vi "ElevatorStateControl.vi"(9 "Elevator State":string) -> (1 "Elevator State Out":string, 2 "Target Elevator Position":dbl, 4 "Target Vacuum Pump Power":dbl)   [LabVIEW 2018]
uses:
  Inputs_DriverStation.vi
  SensorReadings.vi
  RobotStates.vi
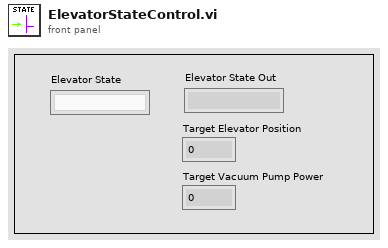
[diagram p1: front panel]
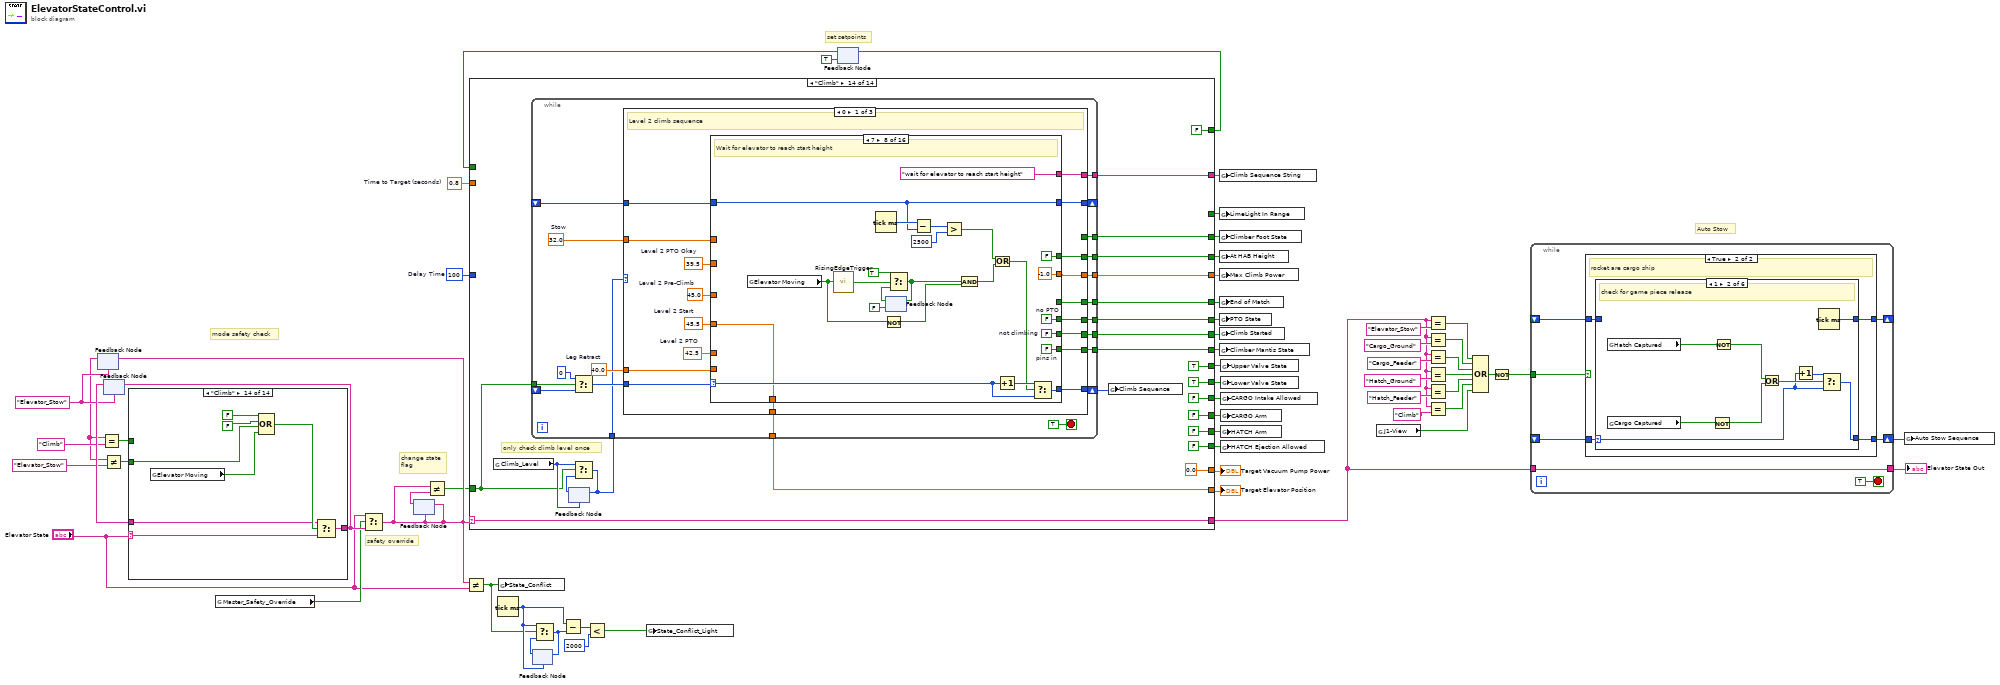
[diagram p0: block diagram]
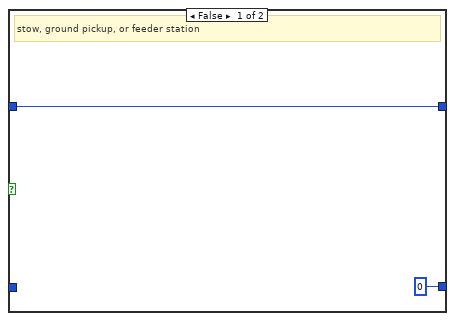
[diagram p2: hidden frame]
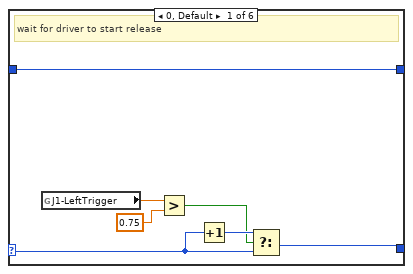
[diagram p3: hidden frame]
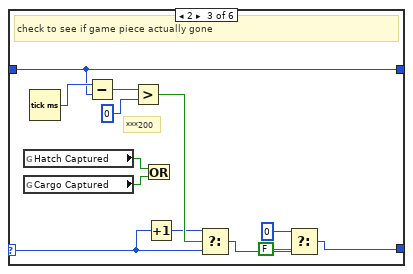
[diagram p4: hidden frame]
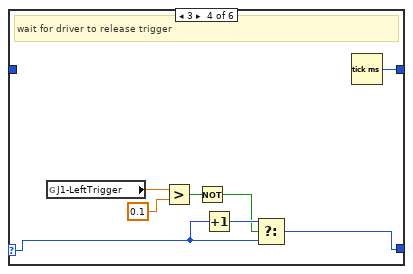
[diagram p5: hidden frame]
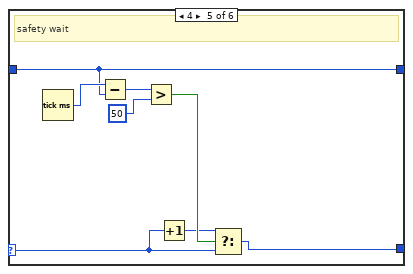
[diagram p6: hidden frame]
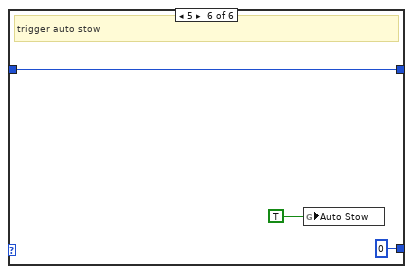
[diagram p7: hidden frame]
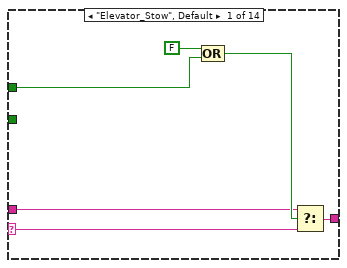
[diagram p8: hidden frame]
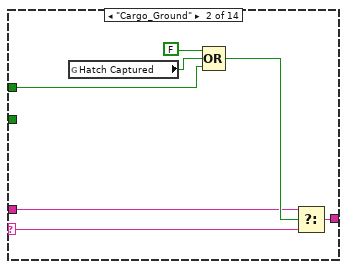
[diagram p9: hidden frame]
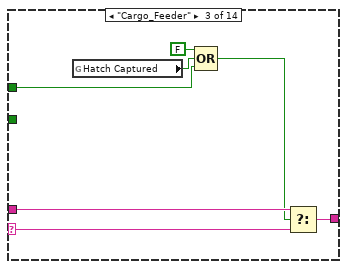
[diagram p10: hidden frame]
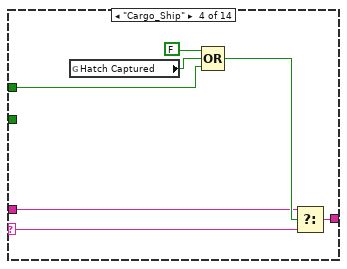
[diagram p11: hidden frame]
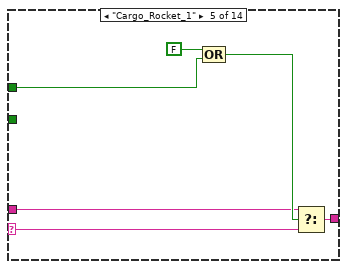
[diagram p12: hidden frame]
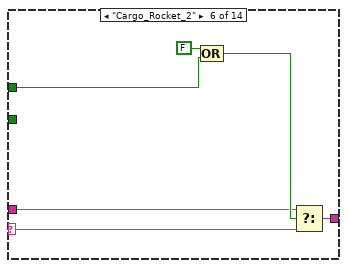
[diagram p13: hidden frame]
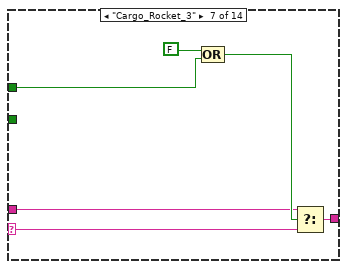
[diagram p14: hidden frame]
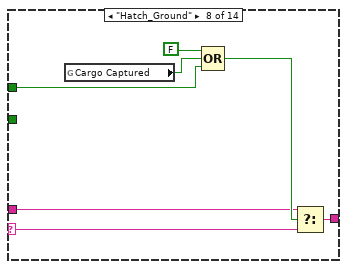
[diagram p15: hidden frame]
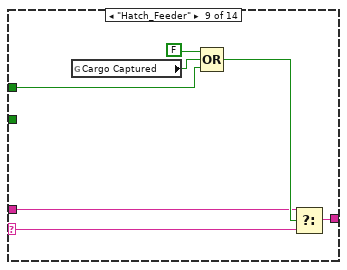
[diagram p16: hidden frame]
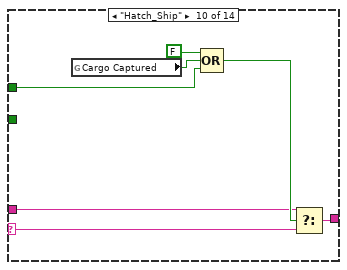
[diagram p17: hidden frame]
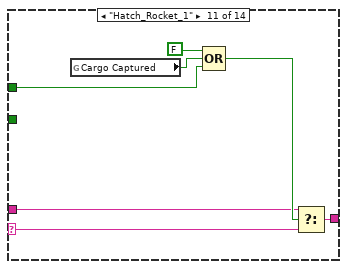
[diagram p18: hidden frame]
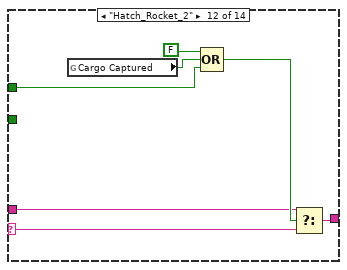
[diagram p19: hidden frame]
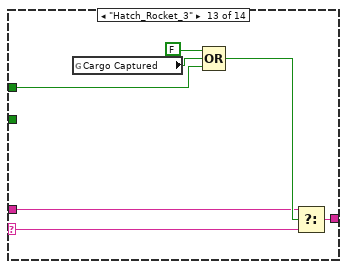
[diagram p20: hidden frame]
diagram:
  w3 = u32 100  # Delay Time
  w4 = 0.8  # Time to Target (seconds)
  w46 = "Elevator_Stow" ("Elevator State")
  # "change state\nflag"
  # "Auto Stow"
  # "safety override"
  # "mode safety check"
  # "set setpoints"
  n1 = feedback #1(w46) -> (w11:string)
  n2 = Equal?(x=w11, y="Climb") -> (x = y?=w47:bool)
  n3 = feedback #2(w46) -> (w49:string)
  n4 = Not Equal?(x=w11, y="Elevator_Stow") -> (x != y?=w10:bool)
  n5 = case shown="\"Climb\"" "Elevator State" {
    selector: "Elevator State" -> [w62 w69 w80 w83 w89 w95 w102 w108 w115 w122 w129 w136 w144 w152]
    tunnel: [w64 w71 w79 w85 w91 w97 w103 w110 w117 w124 w131 w138 w145 w153] -> w54
    tunnel: w49 -> [w63 w70 w78 w84 w90 w96 w101 w109 w116 w123 w130 w137 w143 w151]
    tunnel: w47 -> [w61 w67 w74 w81 w88 w94 w100 w106 w113 w120 w127 w134 w141 _]
    tunnel: w10 -> [_ _ _ _ _ _ _ _ _ _ _ _ _ w150]
    frame "Elevator_Stow", Default {
      n6 = Compound Arithmetic op=OR(FALSE, w61) -> (w65:bool)
      n7 = Select(t=w63, s=w65, f=w62) -> (s? t:f=w64:string)
    }
    frame "Cargo_Ground" {
      n8 = global read "SensorReadings.vi" "Hatch Captured"() -> (w68:bool)
      n9 = Compound Arithmetic op=OR(FALSE, w68, w67) -> (w72:bool)
      n10 = Select(t=w70, s=w72, f=w69) -> (s? t:f=w71:string)
    }
    frame "Cargo_Feeder" {
      n11 = global read "SensorReadings.vi" "Hatch Captured"() -> (w75:bool)
      n12 = Compound Arithmetic op=OR(FALSE, w75, w74) -> (w76:bool)
      n13 = Select(t=w78, s=w76, f=w80) -> (s? t:f=w79:string)
    }
    frame "Cargo_Ship" {
      n14 = global read "SensorReadings.vi" "Hatch Captured"() -> (w82:bool)
      n15 = Compound Arithmetic op=OR(FALSE, w82, w81) -> (w86:bool)
      n16 = Select(t=w84, s=w86, f=w83) -> (s? t:f=w85:string)
    }
    frame "Cargo_Rocket_1" {
      n17 = Compound Arithmetic op=OR(FALSE, w88) -> (w92:bool)
      n18 = Select(t=w90, s=w92, f=w89) -> (s? t:f=w91:string)
    }
    frame "Cargo_Rocket_2" {
      n19 = Compound Arithmetic op=OR(FALSE, w94) -> (w98:bool)
      n20 = Select(t=w96, s=w98, f=w95) -> (s? t:f=w97:string)
    }
    frame "Cargo_Rocket_3" {
      n21 = Compound Arithmetic op=OR(FALSE, w100) -> (w104:bool)
      n22 = Select(t=w101, s=w104, f=w102) -> (s? t:f=w103:string)
    }
    frame "Hatch_Ground" {
      n23 = global read "SensorReadings.vi" "Cargo Captured"() -> (w107:bool)
      n24 = Compound Arithmetic op=OR(FALSE, w107, w106) -> (w111:bool)
      n25 = Select(t=w109, s=w111, f=w108) -> (s? t:f=w110:string)
    }
    frame "Hatch_Feeder" {
      n26 = global read "SensorReadings.vi" "Cargo Captured"() -> (w114:bool)
      n27 = Compound Arithmetic op=OR(FALSE, w114, w113) -> (w118:bool)
      n28 = Select(t=w116, s=w118, f=w115) -> (s? t:f=w117:string)
    }
    frame "Hatch_Ship" {
      n29 = global read "SensorReadings.vi" "Cargo Captured"() -> (w121:bool)
      n30 = Compound Arithmetic op=OR(FALSE, w121, w120) -> (w125:bool)
      n31 = Select(t=w123, s=w125, f=w122) -> (s? t:f=w124:string)
    }
    frame "Hatch_Rocket_1" {
      n32 = global read "SensorReadings.vi" "Cargo Captured"() -> (w128:bool)
      n33 = Compound Arithmetic op=OR(FALSE, w128, w127) -> (w132:bool)
      n34 = Select(t=w130, s=w132, f=w129) -> (s? t:f=w131:string)
    }
    frame "Hatch_Rocket_2" {
      n35 = global read "SensorReadings.vi" "Cargo Captured"() -> (w135:bool)
      n36 = Compound Arithmetic op=OR(FALSE, w135, w134) -> (w139:bool)
      n37 = Select(t=w137, s=w139, f=w136) -> (s? t:f=w138:string)
    }
    frame "Hatch_Rocket_3" {
      n38 = global read "SensorReadings.vi" "Cargo Captured"() -> (w142:bool)
      n39 = Compound Arithmetic op=OR(FALSE, w142, w141) -> (w146:bool)
      n40 = Select(t=w143, s=w146, f=w144) -> (s? t:f=w145:string)
    }
    frame "Climb" {
      n41 = global read "RobotStates.vi" "Elevator Moving"() -> (w149:bool)
      n42 = Compound Arithmetic op=OR(FALSE, FALSE ("Cargo Captured"), w150, w149) -> (w154:bool)
      n43 = Select(t=w151, s=w154, f=w152) -> (s? t:f=w153:string)
    }
  }
  n44 = feedback-in #2(w54) -> ()
  n45 = global read "Inputs_DriverStation.vi" "Master_Safety_Override"() -> (w53:bool)
  n46 = Select(t="Elevator State", s=w53, f=w54) -> (s? t:f=w16:string)
  n47 = feedback-in #1(w16) -> ()
  n48 = feedback-in #3(w16) -> ()
  n49 = feedback #3(w16) -> (w17:string)
  n50 = Not Equal?(x=w16, y=w17) -> (x != y?=w15:bool)
  n51 = Not Equal?(x=w16, y="Elevator State") -> (x != y?=w22:bool)
  n52 = Tick Count (ms)() -> (millisecond timer value=w26:u32)
  n53 = global write "RobotStates.vi" "State_Conflict"(w22) -> ()
  n54 = feedback #4(w26) -> (w27:u32)
  n55 = Select(t=w26, s=w22, f=w27) -> (s? t:f=w25:u32)
  n56 = feedback-in #4(w25) -> ()
  n57 = Subtract(x=w26, y=w25) -> (x-y=w24:u32)
  n58 = Less?(x=w24, y=u32 2000) -> (x < y?=w21:bool)
  n59 = global write "RobotStates.vi" "State_Conflict_Light"(w21) -> ()
  n60 = feedback #5(TRUE) -> (w19:bool)
  n61 = case shown="\"Climb\"" w16 {
    selector: w16 -> [w179 w194 w234 w252 w293 w315 w337 w351 w413 w454 w495 w510 w525 w550]
    tunnel: [FALSE TRUE TRUE TRUE TRUE TRUE TRUE FALSE FALSE FALSE FALSE FALSE FALSE FALSE] -> w60
    tunnel: [w179 w194 w234 w252 w293 w315 w337 w351 w413 w454 w495 w510 w525 w550] -> w29
    tunnel: [w157 FALSE w197 w235 TRUE w296 w319 FALSE FALSE FALSE FALSE FALSE FALSE FALSE] -> w59
    tunnel: [w178 32.0 w204 w236 w279 w300 w317 32.0 w378 w440 w481 61.5 91.0 w536] -> w58
    tunnel: [FALSE FALSE FALSE FALSE FALSE FALSE FALSE TRUE w382 TRUE TRUE TRUE TRUE FALSE] -> w57
    tunnel: [w170 0.0 0.0 0.0 0.0 0.0 0.0 w347 w411 w452 w493 w506 w521 0.0 ("Vacuum_Pump")] -> w55
    tunnel: [FALSE FALSE FALSE FALSE FALSE FALSE FALSE TRUE TRUE TRUE TRUE TRUE TRUE FALSE] -> w56
    tunnel: [TRUE TRUE TRUE TRUE TRUE TRUE TRUE TRUE FALSE FALSE FALSE FALSE FALSE TRUE] -> w52
    tunnel: [TRUE TRUE TRUE TRUE TRUE TRUE TRUE FALSE TRUE TRUE TRUE TRUE TRUE TRUE] -> w51
    tunnel: [FALSE FALSE FALSE FALSE FALSE FALSE FALSE FALSE FALSE FALSE FALSE FALSE FALSE w539] -> w1
    tunnel: [w168 FALSE FALSE FALSE FALSE FALSE FALSE FALSE FALSE FALSE FALSE FALSE FALSE FALSE] -> w20
    tunnel: w19 -> [w164 _ _ _ _ _ _ _ _ _ _ _ _ _]
    tunnel: w15 -> [_ _ w212 _ _ _ _ _ w384 _ _ _ _ w538]
    tunnel: [w167 w184 w203 w244 w284 w307 w329 w342 w390 w447 w488 w501 w516 w535] -> w14
    tunnel: [w166 w183 w202 w243 w283 w306 w328 w341 w389 w446 w487 w500 w515 w534] -> w13
    tunnel: [FALSE FALSE FALSE FALSE FALSE FALSE FALSE FALSE FALSE FALSE FALSE FALSE FALSE w533] -> w9
    tunnel: [_ _ _ _ _ _ _ _ _ _ _ _ _ w531] -> w8
    tunnel: [-1.0 ("y") -1.0 ("y") -1.0 ("y") -1.0 ("y") -1.0 ("y") -1.0 ("y") -1.0 ("y") -1.0 ("y") -1.0 ("y") -1.0 ("y") -1.0 ("y") -1.0 ("y") -1.0 ("y") w530] -> w7
    tunnel: [_ _ _ _ _ _ _ _ _ _ _ _ _ w529] -> w6
    tunnel: [_ _ _ _ w271 _ _ _ w371 w433 w474 _ _ _] -> w5
    tunnel: w4 -> [_ _ _ _ w269 _ _ _ w369 w432 w472 _ _ _]
    tunnel: w3 -> [_ _ _ _ w270 _ _ _ w370 w431 w473 _ _ _]
    tunnel: [_ _ _ _ _ _ _ _ _ _ _ _ _ w528] -> w2
    frame "Elevator_Stow", Default {
      w166 = FALSE  # no PTO
      w167 = FALSE  # not climbing
      w178 = 30.0  # below 34.5 to ensure reset
      n62 = global read "Inputs_DriverStation.vi" "Reinit_Stow_Vacuum"() -> (w161:bool)
      n63 = global read "Inputs_DriverStation.vi" "Vacuum_Pump"() -> (w172:dbl)
      n64 = global read "RobotStates.vi" "Autopilot"() -> (w160:bool)
      n65 = Select(t=TRUE, s=w161, f=w164) -> (s? t:f=w163:bool)
      n66 = Select(t=w172, s=w163, f=0.0) -> (s? t:f=w170:dbl)
      n67 = Select(t=TRUE, s=w163, f=w163) -> (s? t:f=w168:bool)
      n68 = Select(t=TRUE, s=w160, f=FALSE) -> (s? t:f=w157:bool)
    }
    frame "Cargo_Ground" {
      w183 = FALSE  # no PTO
      w184 = FALSE  # not climbing
    }
    frame "Cargo_Feeder" {
      w199 = TRUE  # hold CARGO arm up
      w202 = FALSE  # no PTO
      w203 = FALSE  # not climbing
      w205 = 32.0  # gotten CARGO
      w209 = FALSE  # gotten CARGO
      w221 = -2.0  # (ft/s)
      w208 = 52.0  # getting CARGO
      w210 = TRUE  # getting CARGO
      # "autopilot"
      # "auto protect CARGO"
      n69 = global read "SensorReadings.vi" "EncoderVel_RightDrive"() -> (w225:dbl)
      n70 = global read "SensorReadings.vi" "EncoderVel_LeftDrive"() -> (w226:dbl)
      n71 = global read "SensorReadings.vi" "Cargo Captured"() -> (w219:bool)
      n72 = Add(x=w226, y=w225) -> (x+y=w224:dbl)
      n73 = Divide(x=w224, y=2.0) -> (x/y=w222:dbl)
      n74 = Less?(x=w222, y=w221) -> (x < y?=w220:bool)
      n75 = And(x=w220, y=w219) -> (x .and. y?=w218:bool)
      n76 = feedback #6(FALSE) -> (w216:bool)
      n77 = Select(t=TRUE, s=w218, f=w216) -> (s? t:f=w214:bool)
      n78 = Select(t=FALSE, s=w212, f=w214) -> (s? t:f=w207:bool)
      n79 = feedback-in #6(w207) -> ()
      n80 = Not(x=w207) -> (.not. x?=w206:bool)
      n81 = global read "RobotStates.vi" "Autopilot"() -> (w200:bool)
      n82 = Select(t=w210, s=w206, f=w209) -> (s? t:f=w198:bool)
      n83 = Select(t=w199, s=w200, f=w198) -> (s? t:f=w197:bool)
      n84 = Select(t=w208, s=w206, f=w205) -> (s? t:f=w204:dbl)
    }
    frame "Cargo_Ship" {
      w243 = FALSE  # no PTO
      w244 = FALSE  # not climbing
      w236 = 48.0
      # "46"
      n85 = global read "SensorReadings.vi" "EncoderPos_Elevator"() -> (w240:dbl)
      n86 = Subtract(x=w240, y=w236) -> (x-y=w239:dbl)
      n87 = Absolute Value(x=w239) -> (abs(x)=w237:dbl)
      n88 = Less?(x=w237, y=5.0) -> (x < y?=w235:bool)
    }
    frame "Cargo_Rocket_1" {
      w260 = 3.0  # feet per second
      w283 = FALSE  # no PTO
      w284 = FALSE  # not climbing
      n89 = global read "SensorReadings.vi" "LimeLight Distance (in)"() -> (w258:dbl)
      n90 = global read "SensorReadings.vi" "EncoderVel_RightDrive"() -> (w267:dbl)
      n91 = global read "SensorReadings.vi" "EncoderVel_LeftDrive"() -> (w268:dbl)
      n92 = Add(x=w268, y=w267) -> (x+y=w266:dbl)
      n93 = Divide(x=w258, y=12.0) -> (x/y=w256:dbl)
      n94 = Divide(x=w266, y=2.0) -> (x/y=w261:dbl)
      n95 = In Range and Coerce(upper limit=10.0, x=w261, lower limit=w260) -> (coerced(x)=w259:dbl)  [unwired: 1 out]
      n96 = Divide(x=w256, y=w259) -> (x/y=w263:dbl)
      n97 = Greater Than 0?(x=w263) -> (x > 0?=w264:bool)
      n98 = Select(t=w263, s=w264, f=inf) -> (s? t:f=w255:dbl)
      n99 = global read "SensorReadings.vi" "LimeLight Valid"() -> (w274:bool)
      n100 = Select(t=w255, s=w274, f=inf) -> (s? t:f=w273:dbl)
      n101 = call "TimeBelowThreshold.vi"("Current Value"=w273, "Threshold"=w269) -> ("Time Below"=w275:u32)  [unwired: 3 in]
      n102 = global read "RobotStates.vi" "Autopilot"() -> (w281:bool)
      n103 = Greater?(x=w275, y=w270) -> (0:w276:bool)
      n104 = call "RisingEdgeTrigger.vi"("Raw Signal"=w276) -> ("Trigger"=w271:bool)
      n105 = Select(t=45.0, s=w281, f=32.0) -> (s? t:f=w279:dbl)
    }
    frame "Cargo_Rocket_2" {
      w306 = FALSE  # no PTO
      w307 = FALSE  # not climbing
      w300 = 62.5
      n106 = global read "SensorReadings.vi" "EncoderPos_Elevator"() -> (w301:dbl)
      n107 = Subtract(x=w301, y=w300) -> (x-y=w299:dbl)
      n108 = Absolute Value(x=w299) -> (abs(x)=w295:dbl)
      n109 = Less?(x=w295, y=10.0) -> (x < y?=w297:bool)
      n110 = Select(t=TRUE, s=w297, f=FALSE) -> (s? t:f=w296:bool)
    }
    frame "Cargo_Rocket_3" {
      w328 = FALSE  # no PTO
      w329 = FALSE  # not climbing
      w317 = 91.0
      n111 = global read "SensorReadings.vi" "EncoderPos_Elevator"() -> (w323:dbl)
      n112 = Subtract(x=w323, y=w317) -> (x-y=w322:dbl)
      n113 = Absolute Value(x=w322) -> (abs(x)=w320:dbl)
      n114 = Less?(x=w320, y=10.0) -> (x < y?=w321:bool)
      n115 = Select(t=TRUE, s=w321, f=FALSE) -> (s? t:f=w319:bool)
    }
    frame "Hatch_Ground" {
      w341 = FALSE  # no PTO
      w342 = FALSE  # not climbing
      n116 = global read "Inputs_DriverStation.vi" "Vacuum_Pump"() -> (w347:dbl)
    }
    frame "Hatch_Feeder" {
      w359 = 3.0  # feet per second
      w389 = FALSE  # no PTO
      w390 = FALSE  # not climbing
      w400 = -2.0  # (ft/s)
      w392 = FALSE  # gotten HATCH
      w406 = TRUE  # to get HATCH
      # "auto protect HATCH"
      n117 = global read "SensorReadings.vi" "EncoderVel_RightDrive"() -> (w404:dbl)
      n118 = global read "SensorReadings.vi" "EncoderVel_LeftDrive"() -> (w405:dbl)
      n119 = global read "SensorReadings.vi" "LimeLight Distance (in)"() -> (w357:dbl)
      n120 = global read "SensorReadings.vi" "EncoderVel_RightDrive"() -> (w367:dbl)
      n121 = global read "SensorReadings.vi" "EncoderVel_LeftDrive"() -> (w368:dbl)
      n122 = global read "SensorReadings.vi" "Hatch Captured"() -> (w386:bool)
      n123 = Add(x=w405, y=w404) -> (x+y=w403:dbl)
      n124 = Divide(x=w403, y=2.0) -> (x/y=w401:dbl)
      n125 = Less?(x=w401, y=w400) -> (x < y?=w399:bool)
      n126 = Add(x=w368, y=w367) -> (x+y=w366:dbl)
      n127 = And(x=w399, y=w386) -> (x .and. y?=w398:bool)
      n128 = Not(x=w386) -> (.not. x?=w385:bool)
      n129 = Divide(x=w357, y=12.0) -> (x/y=w355:dbl)
      n130 = Divide(x=w366, y=2.0) -> (x/y=w360:dbl)
      n131 = Or(x=w385, y=w384) -> (x .or. y?=w383:bool)
      n132 = feedback #7(FALSE) -> (w396:bool)
      n133 = Select(t=TRUE, s=w398, f=w396) -> (s? t:f=w394:bool)
      n134 = In Range and Coerce(upper limit=10.0 ("feet per second"), x=w360, lower limit=w359) -> (coerced(x)=w358:dbl)  [unwired: 1 out]
      n135 = Select(t=FALSE, s=w383, f=w394) -> (s? t:f=w391:bool)
      n136 = feedback-in #7(w391) -> ()
      n137 = Divide(x=w355, y=w358) -> (x/y=w363:dbl)
      n138 = Not(x=w391) -> (.not. x?=w387:bool)
      n139 = Greater Than 0?(x=w363) -> (x > 0?=w364:bool)
      n140 = Select(t=w363, s=w364, f=inf) -> (s? t:f=w361:dbl)
      n141 = global read "SensorReadings.vi" "LimeLight Valid"() -> (w375:bool)
      n142 = Select(t=w406, s=w387, f=w392) -> (s? t:f=w382:bool)
      n143 = Select(t=w361, s=w375, f=inf) -> (s? t:f=w376:dbl)
      n144 = global read "RobotStates.vi" "Autopilot"() -> (w381:bool)
      n145 = call "TimeBelowThreshold.vi"("Current Value"=w376, "Threshold"=w369) -> ("Time Below"=w373:u32)  [unwired: 3 in]
      n146 = global read "Inputs_DriverStation.vi" "Vacuum_Pump"() -> (w411:dbl)
      n147 = Greater?(x=w373, y=w370) -> (0:w372:bool)
      n148 = Select(t=55.0, s=w381, f=32.0) -> (s? t:f=w378:dbl)
      n149 = call "RisingEdgeTrigger.vi"("Raw Signal"=w372) -> ("Trigger"=w371:bool)
    }
    frame "Hatch_Ship" {
      w422 = 3.0  # feet per second
      w446 = FALSE  # no PTO
      w447 = FALSE  # not climbing
      n150 = global read "SensorReadings.vi" "LimeLight Distance (in)"() -> (w420:dbl)
      n151 = global read "SensorReadings.vi" "EncoderVel_RightDrive"() -> (w429:dbl)
      n152 = global read "SensorReadings.vi" "EncoderVel_LeftDrive"() -> (w430:dbl)
      n153 = Add(x=w430, y=w429) -> (x+y=w428:dbl)
      n154 = Divide(x=w420, y=12.0) -> (x/y=w418:dbl)
      n155 = Divide(x=w428, y=2.0) -> (x/y=w423:dbl)
      n156 = In Range and Coerce(upper limit=10.0, x=w423, lower limit=w422) -> (coerced(x)=w421:dbl)  [unwired: 1 out]
      n157 = Divide(x=w418, y=w421) -> (x/y=w425:dbl)
      n158 = Greater Than 0?(x=w425) -> (x > 0?=w426:bool)
      n159 = Select(t=w425, s=w426, f=inf) -> (s? t:f=w417:dbl)
      n160 = global read "SensorReadings.vi" "LimeLight Valid"() -> (w437:bool)
      n161 = Select(t=w417, s=w437, f=inf) -> (s? t:f=w438:dbl)
      n162 = call "TimeBelowThreshold.vi"("Current Value"=w438, "Threshold"=w432) -> ("Time Below"=w435:u32)  [unwired: 3 in]
      n163 = global read "RobotStates.vi" "Autopilot"() -> (w443:bool)
      n164 = global read "Inputs_DriverStation.vi" "Vacuum_Pump"() -> (w452:dbl)
      n165 = Greater?(x=w435, y=w431) -> (0:w434:bool)
      n166 = call "RisingEdgeTrigger.vi"("Raw Signal"=w434) -> ("Trigger"=w433:bool)
      n167 = Select(t=55.0, s=w443, f=32.0) -> (s? t:f=w440:dbl)
    }
    frame "Hatch_Rocket_1" {
      w463 = 3.0  # feet per second
      w487 = FALSE  # no PTO
      w488 = FALSE  # not climbing
      # "autopilot"
      n168 = global read "SensorReadings.vi" "LimeLight Distance (in)"() -> (w461:dbl)
      n169 = global read "SensorReadings.vi" "EncoderVel_RightDrive"() -> (w470:dbl)
      n170 = global read "SensorReadings.vi" "EncoderVel_LeftDrive"() -> (w471:dbl)
      n171 = Add(x=w471, y=w470) -> (x+y=w469:dbl)
      n172 = Divide(x=w461, y=12.0) -> (x/y=w459:dbl)
      n173 = Divide(x=w469, y=2.0) -> (x/y=w464:dbl)
      n174 = In Range and Coerce(upper limit=10.0, x=w464, lower limit=w463) -> (coerced(x)=w462:dbl)  [unwired: 1 out]
      n175 = Divide(x=w459, y=w462) -> (x/y=w466:dbl)
      n176 = Greater Than 0?(x=w466) -> (x > 0?=w467:bool)
      n177 = Select(t=w466, s=w467, f=inf) -> (s? t:f=w458:dbl)
      n178 = global read "SensorReadings.vi" "LimeLight Valid"() -> (w477:bool)
      n179 = Select(t=w458, s=w477, f=inf) -> (s? t:f=w476:dbl)
      n180 = call "TimeBelowThreshold.vi"("Current Value"=w476, "Threshold"=w472) -> ("Time Below"=w478:u32)  [unwired: 3 in]
      n181 = Greater?(x=w478, y=w473) -> (0:w479:bool)
      n182 = global read "RobotStates.vi" "Autopilot"() -> (w484:bool)
      n183 = global read "Inputs_DriverStation.vi" "Vacuum_Pump"() -> (w493:dbl)
      n184 = call "RisingEdgeTrigger.vi"("Raw Signal"=w479) -> ("Trigger"=w474:bool)
      n185 = Select(t=55.0, s=w484, f=32.0) -> (s? t:f=w481:dbl)
    }
    frame "Hatch_Rocket_2" {
      w500 = FALSE  # no PTO
      w501 = FALSE  # not climbing
      n186 = global read "Inputs_DriverStation.vi" "Vacuum_Pump"() -> (w506:dbl)
    }
    frame "Hatch_Rocket_3" {
      w515 = FALSE  # no PTO
      w516 = FALSE  # not climbing
      n187 = global read "Inputs_DriverStation.vi" "Vacuum_Pump"() -> (w521:dbl)
    }
    frame "Climb" {
      # "only check climb level once"
      n188 = global read "Inputs_DriverStation.vi" "Climb_Level"() -> (w540:u8)
      n189 = feedback #8(w540) -> (w541:u8)
      n190 = Select(t=w540, s=w538, f=w541) -> (s? t:f=w537:u8)
      n191 = while {
        shift-right: [w569] -> w532
        shift-left: _ -> [w565]
        shift-right: [w568] -> _
        shift-left: _ -> [w567]
        tunnel: [w566] -> w539
        tunnel: w538 -> [w563]
        tunnel: w537 -> [w556]
        tunnel: [w558] -> w536
        tunnel: [w561] -> w535
        tunnel: [w560] -> w534
        tunnel: [w559] -> w533
        tunnel: [w555] -> w531
        tunnel: [w554] -> w530
        tunnel: [w553] -> w529
        tunnel: [w551] -> w528
        stop <- TRUE stop-if-true
        w552 = 32.0  # Stow
        w557 = 40.0  # Leg Retract
        n192 = Select(t=0, s=w563, f=w565) -> (s? t:f=w564:i32)
        n193 = case shown="0" w556 {
          tunnel: [w582 w846 w1069] -> w569
          tunnel: [w586 w853 w1076] -> w568
          tunnel: w567 -> [w588 w854 w1077]
          tunnel: [w581 w847 w1070] -> w566
          tunnel: w564 -> [w584 w852 w1075]
          tunnel: [w579 w848 w1071] -> w561
          tunnel: [w580 w849 w1072] -> w560
          tunnel: [w583 w850 w1073] -> w559
          tunnel: [w578 w845 w1068] -> w558
          tunnel: w557 -> [w585 w851 w1074]
          tunnel: [w587 w844 w1067] -> w555
          tunnel: [w577 w842 w1065] -> w554
          tunnel: [w576 w840 w1063] -> w553
          tunnel: w552 -> [w571 w839 w1062]
          tunnel: [_ _ w1061] -> w551
          frame 0 {
            w575 = 45.0  # Level 2 Pre-Climb
            w572 = 39.5  # Level 2 PTO Okay
            w574 = 45.5  # Level 2 Start
            w573 = 42.5  # Level 2 PTO
            # "Level 2 climb sequence"
            n194 = case shown="7" w584 {
              selector: w584 -> [w598 w614 w634 w651 w662 w683 w695 w719 w737 w748 w766 w775 w790 w802 w819 w833]
              tunnel: [w600 w616 w630 w650 w661 w682 w696 w720 w736 w747 w765 w774 w789 w801 w818 w833] -> w582
              tunnel: [w597 w601 w620 w648 w664 w675 w686 w706 w732 w740 w753 w778 w792 w804 w826 w836] -> w586
              tunnel: w588 -> [_ w604 w620 _ w664 w675 _ w706 w732 _ w753 w778 w792 w804 w826 w836]
              tunnel: [w596 w613 w640 w649 w660 w685 w699 w723 w739 w750 w768 w779 w793 w805 w827 w837] -> w581
              tunnel: [w589 w602 w624 w641 w653 w668 _ w710 _ _ _ _ w785 w800 w821 w830] -> w578
              tunnel: [w594 w612 w629 w646 w659 w678 w700 w724 w735 w746 w764 w780 w794 w806 w828 w838] -> w579
              tunnel: [w593 w611 w628 w645 w658 w677 w701 w725 w734 w745 w763 w773 w788 w798 w824 w834] -> w580
              tunnel: [FALSE FALSE FALSE FALSE FALSE FALSE FALSE FALSE FALSE FALSE FALSE w777 TRUE TRUE TRUE FALSE] -> w583
              tunnel: w585 -> [_ _ _ _ _ _ _ _ _ _ _ _ w785 w800 w821 w830]
              tunnel: ["release mantis" "wait for mantis to deploy" "wait for elevator to reach climb height" "lock mantis" "confirm mantis lock" "wait for the driver to start climbing #1" "wait for driver to raise elevator" "wait for elevator to reach start height" "wait for elevator to pass PTO height" "engage the PTO" "ensure PTO is engaged" "wait for the robot to be on HAB" "stop climbing" "wait to disengage PTO" "retract the legs after confirm " "elevator powered down"] -> w587
              tunnel: [-1.0 ("y") -1.0 ("y") -1.0 ("y") -1.0 ("y") -1.0 ("y") -1.0 ("y") -1.0 ("y") -1.0 ("y") -0.05 ("y") -0.05 ("y") -0.05 ("y") -1.0 ("y") -1.0 ("y") -1.0 ("y") -1.0 ("y") -1.0 ("y")] -> w577
              tunnel: [_ _ _ _ _ _ _ _ _ _ _ _ _ _ _ w829] -> w576
              tunnel: w575 -> [_ _ w624 w641 w653 w668 _ _ _ _ _ _ _ _ _ _]
              tunnel: w574 -> [_ _ _ _ _ _ _ w710 _ _ _ _ _ _ _ _]
              tunnel: w573 -> [_ _ _ _ _ _ _ _ w727 _ _ _ _ _ _ _]
              tunnel: w572 -> [_ _ _ _ _ _ _ _ _ _ w751 _ _ _ _ _]
              tunnel: w571 -> [w589 w602 _ _ _ _ _ _ _ _ _ _ _ _ _ _]
              frame 0, Default {
                w593 = FALSE  # no PTO
                w594 = FALSE  # not climbing
                w596 = TRUE  # pins out
                # "release mantis pins and command to climb height"
                n195 = Increment(x=w598) -> (x+1=w599:i32)
                n196 = Select(t=w599, s=TRUE, f=w598) -> (s? t:f=w600:i32)
                n197 = Tick Count (ms)() -> (millisecond timer value=w597:u32)
              }
              frame 1 {
                w611 = FALSE  # no PTO
                w612 = FALSE  # not climbing
                w613 = TRUE  # pins out
                # "wait for mantis to deploy"
                n198 = Tick Count (ms)() -> (millisecond timer value=w607:u32)
                n199 = Subtract(x=w607, y=w604) -> (x-y=w606:u32)
                n200 = Greater?(x=w606, y=u32 0) -> (0:w603:bool)
                n201 = Increment(x=w614) -> (x+1=w615:i32)
                n202 = Select(t=w615, s=w603, f=w614) -> (s? t:f=w616:i32)
                n203 = Tick Count (ms)() -> (millisecond timer value=w601:u32)
              }
              frame 2 {
                w628 = FALSE  # no PTO
                w629 = FALSE  # not climbing
                w640 = TRUE  # pins out
                # "wait for elevator to start moving\nand then stop moving"
                # "wait for elevator to reach climb position"
                n204 = global read "RobotStates.vi" "Elevator Moving"() -> (w632:bool)
                n205 = call "RisingEdgeTrigger.vi"("Raw Signal"=w632) -> ("Trigger"=w639:bool)
                n206 = Tick Count (ms)() -> (millisecond timer value=w623:u32)
                n207 = Not(x=w632) -> (.not. x?=w631:bool)
                n208 = feedback #9(FALSE) -> (w637:bool)
                n209 = Select(t=TRUE, s=w639, f=w637) -> (s? t:f=w633:bool)
                n210 = feedback-in #9(w633) -> ()
                n211 = Subtract(x=w623, y=w620) -> (x-y=w622:u32)
                n212 = Greater?(x=w622, y=u32 2500) -> (0:w617:bool)
                n213 = And(x=w633, y=w631) -> (x .and. y?=w619:bool)
                n214 = Or(x=w617, y=w619) -> (x .or. y?=w618:bool)
                n215 = Increment(x=w634) -> (x+1=w635:i32)
                n216 = Select(t=w635, s=w618, f=w634) -> (s? t:f=w630:i32)
              }
              frame 3 {
                w645 = FALSE  # no PTO
                w646 = FALSE  # not climbing
                w649 = FALSE  # pins in
                # "lock mantis pins"
                n217 = Increment(x=w651) -> (x+1=w652:i32)
                n218 = Tick Count (ms)() -> (millisecond timer value=w648:u32)
                n219 = Select(t=w652, s=TRUE, f=w651) -> (s? t:f=w650:i32)
              }
              frame 4 {
                w658 = FALSE  # no PTO
                w659 = FALSE  # not climbing
                w660 = FALSE  # pins in
                # "wait for mantis legs to lock"
                n220 = Tick Count (ms)() -> (millisecond timer value=w667:u32)
                n221 = Subtract(x=w667, y=w664) -> (x-y=w666:u32)
                n222 = Greater?(x=w666, y=u32 500) -> (0:w656:bool)
                n223 = Increment(x=w662) -> (x+1=w663:i32)
                n224 = Select(t=w663, s=w656, f=w662) -> (s? t:f=w661:i32)
              }
              frame 5 {
                w677 = FALSE  # no PTO
                w678 = FALSE  # not climbing
                w685 = FALSE  # pins in
                # "wait for the driver to start climbing"
                n225 = global read "Inputs_DriverStation.vi" "J1-RightTrigger"() -> (w674:dbl)
                n226 = Greater?(x=w674, y=0.2) -> (0:w672:bool)
                n227 = feedback #10(FALSE) -> (w679:bool)
                n228 = Select(t=TRUE, s=w672, f=w679) -> (s? t:f=w671:bool)
                n229 = feedback-in #10(w671) -> ()
                n230 = Increment(x=w683) -> (x+1=w684:i32)
                n231 = Select(t=w684, s=w671, f=w683) -> (s? t:f=w682:i32)
              }
              frame 6 {
                w701 = FALSE  # no PTO
                w700 = TRUE  # climbing
                w699 = FALSE  # pins in
                # "Lower elevator contacts HAB first time"
                n232 = global read "Inputs_DriverStation.vi" "J1-LeftTrigger"() -> (w691:dbl)
                n233 = Greater?(x=w691, y=0.75) -> (0:w689:bool)
                n234 = feedback #11(FALSE) -> (w692:bool)
                n235 = Select(t=TRUE, s=w689, f=w692) -> (s? t:f=w688:bool)
                n236 = feedback-in #11(w688) -> ()
                n237 = Tick Count (ms)() -> (millisecond timer value=w686:u32)
                n238 = Increment(x=w695) -> (x+1=w697:i32)
                n239 = Select(t=w697, s=w688, f=w695) -> (s? t:f=w696:i32)
              }
              frame 7 {
                w725 = FALSE  # no PTO
                w724 = FALSE  # not climbing
                w723 = FALSE  # pins in
                # "Wait for elevator to reach start height"
                n240 = global read "RobotStates.vi" "Elevator Moving"() -> (w712:bool)
                n241 = call "RisingEdgeTrigger.vi"("Raw Signal"=w712) -> ("Trigger"=w717:bool)
                n242 = Tick Count (ms)() -> (millisecond timer value=w709:u32)
                n243 = Not(x=w712) -> (.not. x?=w711:bool)
                n244 = feedback #12(FALSE) -> (w715:bool)
                n245 = Select(t=TRUE, s=w717, f=w715) -> (s? t:f=w713:bool)
                n246 = feedback-in #12(w713) -> ()
                n247 = Subtract(x=w709, y=w706) -> (x-y=w708:u32)
                n248 = Greater?(x=w708, y=u32 2500) -> (0:w705:bool)
                n249 = And(x=w713, y=w711) -> (x .and. y?=w704:bool)
                n250 = Or(x=w705, y=w704) -> (x .or. y?=w703:bool)
                n251 = Increment(x=w719) -> (x+1=w721:i32)
                n252 = Select(t=w721, s=w703, f=w719) -> (s? t:f=w720:i32)
              }
              frame 8 {
                w734 = FALSE  # no PTO
                w735 = TRUE  # climbing
                w739 = FALSE  # pins in
                # "wait for elevator to pass PTO height"
                n253 = global read "SensorReadings.vi" "EncoderPos_Elevator"() -> (w728:dbl)
                n254 = Less Or Equal?(x=w728, y=w727) -> (x <= y?=w729:bool)
                n255 = Increment(x=w737) -> (x+1=w738:i32)
                n256 = Select(t=w738, s=w729, f=w737) -> (s? t:f=w736:i32)
              }
              frame 9 {
                w745 = TRUE  # PTO
                w746 = TRUE  # climbing
                w750 = FALSE  # pins in
                # "engage the PTO"
                n257 = Increment(x=w748) -> (x+1=w749:i32)
                n258 = Tick Count (ms)() -> (millisecond timer value=w740:u32)
                n259 = Select(t=w749, s=TRUE, f=w748) -> (s? t:f=w747:i32)
              }
              frame 10 {
                w763 = TRUE  # PTO
                w764 = TRUE  # climbing
                w768 = FALSE  # pins in
                # "timeout"
                # "ensure PTO is engaged"
                n260 = global read "SensorReadings.vi" "EncoderPos_Elevator"() -> (w759:dbl)
                n261 = Tick Count (ms)() -> (millisecond timer value=w756:u32)
                n262 = Less Or Equal?(x=w759, y=w751) -> (x <= y?=w758:bool)
                n263 = Subtract(x=w756, y=w753) -> (x-y=w755:u32)
                n264 = Greater?(x=w755, y=u32 1000) -> (0:w752:bool)
                n265 = Or(x=w752, y=w758) -> (x .or. y?=w757:bool)
                n266 = Increment(x=w766) -> (x+1=w767:i32)
                n267 = Select(t=w767, s=w757, f=w766) -> (s? t:f=w765:i32)
              }
              frame 11 {
                w773 = TRUE  # PTO
                w780 = TRUE  # climbing
                w779 = FALSE  # pins in
                # "wait for robot to be secure on HAB"
                n268 = global read "Inputs_DriverStation.vi" "Master_Safety_Override"() -> (w781:bool)
                n269 = global read "SensorReadings.vi" "Robot On Ground"() -> (w769:bool)
                n270 = global read "Inputs_DriverStation.vi" "J1-Menu"() -> (w782:bool)
                n271 = Or(x=w769, y=w781) -> (x .or. y?=w777:bool)
                n272 = And(x=w782, y=w777) -> (x .and. y?=w772:bool)
                n273 = Increment(x=w775) -> (x+1=w776:i32)
                n274 = Select(t=w776, s=w772, f=w775) -> (s? t:f=w774:i32)
              }
              frame 12 {
                w788 = TRUE  # PTO
                w794 = FALSE  # not climbing
                w793 = FALSE  # pins in
                # "stop \"climbing\""
                n275 = Increment(x=w790) -> (x+1=w791:i32)
                n276 = Select(t=w791, s=TRUE, f=w790) -> (s? t:f=w789:i32)
              }
              frame 13 {
                w798 = TRUE  # PTO
                w806 = FALSE  # not climbing
                w805 = FALSE  # pins in
                # "wait to disengage PTO"
                n277 = Increment(x=w802) -> (x+1=w803:i32)
                n278 = Select(t=w803, s=TRUE, f=w802) -> (s? t:f=w801:i32)
              }
              frame 14 {
                w824 = FALSE  # no PTO
                w828 = FALSE  # not climbing
                w827 = FALSE  # pins in
                # "retract legs"
                n279 = global read "Inputs_DriverStation.vi" "J1-Menu"() -> (w808:bool)
                n280 = Not(x=w808) -> (.not. x?=w809:bool)
                n281 = feedback #13(FALSE ("PTO")) -> (w812:bool)
                n282 = Select(t=TRUE ("no PTO"), s=w809, f=w812) -> (s? t:f=w807:bool)
                n283 = feedback-in #13(w807) -> ()
                n284 = And(x=w807, y=w808) -> (x .and. y?=w810:bool)
                n285 = feedback #14(FALSE ("PTO")) -> (w816:bool)
                n286 = Select(t=TRUE ("no PTO"), s=w810, f=w816) -> (s? t:f=w814:bool)
                n287 = feedback-in #14(w814) -> ()
                n288 = Increment(x=w819) -> (x+1=w820:i32)
                n289 = Select(t=w820, s=w814, f=w819) -> (s? t:f=w818:i32)
              }
              frame 15 {
                w829 = TRUE  # end of match
                w834 = FALSE  # no PTO
                w838 = FALSE  # not climbing
                w837 = FALSE  # pins in
                # "turn off the elevator"
              }
            }
          }
          frame 1, Default {
            w841 = 57.0  # Level 3 PTO Okay
            w843 = 62.0  # Level 3 Start
            w855 = 60.0  # Level 3 PTO
            # "Level 3 climb sequence"
            n290 = case shown="3" w852 {
              selector: w852 -> [w865 w880 w895 w912 w923 w944 w957 w969 w988 w997 w1012 w1024 w1041 w1055]
              tunnel: [w867 w882 w890 w911 w922 w943 w956 w968 w987 w996 w1011 w1023 w1040 w1055] -> w846
              tunnel: [w864 w870 w888 w909 w925 w936 w952 w960 w973 w1000 w1014 w1026 w1048 w1058] -> w853
              tunnel: w854 -> [_ w870 w888 _ w925 w936 w952 _ w973 w1000 w1014 w1026 w1048 w1058]
              tunnel: [w863 w879 w901 w910 w921 w946 w959 w971 w990 w1001 w1015 w1027 w1049 w1059] -> w847
              tunnel: [w856 w868 w884 w903 w915 w930 _ w963 w983 _ w1007 w1022 w1043 w1052] -> w845
              tunnel: w855 -> [_ _ _ _ _ _ w949 w963 w983 _ _ _ _ _]
              tunnel: [w861 w878 w889 w907 w920 w939 w955 w967 w986 w1002 w1016 w1028 w1050 w1060] -> w848
              tunnel: [w860 w877 w887 w906 w919 w938 w954 w966 w985 w995 w1010 w1020 w1046 w1056] -> w849
              tunnel: [FALSE FALSE FALSE FALSE FALSE FALSE FALSE FALSE FALSE w999 TRUE TRUE TRUE FALSE] -> w850
              tunnel: w851 -> [_ _ _ _ _ _ _ _ _ _ w1007 w1022 w1043 w1052]
              tunnel: ["release mantis" "wait for mantis to deploy" "wait for elevator to reach climb height" "lock mantis" "confirm mantis lock" "wait for the driver to start climbing" "wait for elevator to pass PTO height" "engage the PTO" "ensure PTO is engaged" "wait for the robot to be on HAB" "stop climbing" "wait to disengage PTO" "retract the legs after confirm " "elevator powered down"] -> w844
              tunnel: w843 -> [_ _ w884 w903 w915 w930 _ _ _ _ _ _ _ _]
              tunnel: [-1.0 ("y") -1.0 ("y") -1.0 ("y") -1.0 ("y") -1.0 ("y") -1.0 ("y") -0.05 ("y") -0.05 ("y") -0.05 ("y") -1.0 ("y") -1.0 ("y") -1.0 ("y") -1.0 ("y") -1.0 ("y")] -> w842
              tunnel: w841 -> [_ _ _ _ _ _ _ _ w979 _ _ _ _ _]
              tunnel: [_ _ _ _ _ _ _ _ _ _ _ _ _ w1051] -> w840
              tunnel: w839 -> [w856 w868 _ _ _ _ _ _ _ _ _ _ _ _]
              frame 0, Default {
                w860 = FALSE  # no PTO
                w861 = FALSE  # not climbing
                w863 = TRUE  # pins out
                # "release mantis pins and command to climb height"
                n291 = Increment(x=w865) -> (x+1=w866:i32)
                n292 = Select(t=w866, s=TRUE, f=w865) -> (s? t:f=w867:i32)
                n293 = Tick Count (ms)() -> (millisecond timer value=w864:u32)
              }
              frame 1 {
                w877 = FALSE  # no PTO
                w878 = FALSE  # not climbing
                w879 = TRUE  # pins out
                # "wait for mantis to deploy"
                n294 = Tick Count (ms)() -> (millisecond timer value=w873:u32)
                n295 = Subtract(x=w873, y=w870) -> (x-y=w872:u32)
                n296 = Greater?(x=w872, y=u32 250) -> (0:w869:bool)
                n297 = Increment(x=w880) -> (x+1=w881:i32)
                n298 = Select(t=w881, s=w869, f=w880) -> (s? t:f=w882:i32)
              }
              frame 2 {
                w887 = FALSE  # no PTO
                w889 = FALSE  # not climbing
                w901 = TRUE  # pins out
                # "wait for elevator to start moving\nand then stop moving"
                # "wait for elevator to reach climb position"
                n299 = global read "RobotStates.vi" "Elevator Moving"() -> (w893:bool)
                n300 = call "RisingEdgeTrigger.vi"("Raw Signal"=w893) -> ("Trigger"=w900:bool)
                n301 = Not(x=w893) -> (.not. x?=w892:bool)
                n302 = feedback #15(FALSE) -> (w898:bool)
                n303 = Select(t=TRUE, s=w900, f=w898) -> (s? t:f=w894:bool)
                n304 = feedback-in #15(w894) -> ()
                n305 = And(x=w894, y=w892) -> (x .and. y?=w891:bool)
                n306 = Increment(x=w895) -> (x+1=w896:i32)
                n307 = Select(t=w896, s=w891, f=w895) -> (s? t:f=w890:i32)
              }
              frame 3 {
                w906 = FALSE  # no PTO
                w907 = FALSE  # not climbing
                w910 = FALSE  # pins in
                # "lock mantis pins"
                n308 = Increment(x=w912) -> (x+1=w913:i32)
                n309 = Tick Count (ms)() -> (millisecond timer value=w909:u32)
                n310 = Select(t=w913, s=TRUE, f=w912) -> (s? t:f=w911:i32)
              }
              frame 4 {
                w919 = FALSE  # no PTO
                w920 = FALSE  # not climbing
                w921 = FALSE  # pins in
                # "wait for mantis legs to lock"
                n311 = Tick Count (ms)() -> (millisecond timer value=w928:u32)
                n312 = Subtract(x=w928, y=w925) -> (x-y=w927:u32)
                n313 = Greater?(x=w927, y=u32 500) -> (0:w917:bool)
                n314 = Increment(x=w923) -> (x+1=w924:i32)
                n315 = Select(t=w924, s=w917, f=w923) -> (s? t:f=w922:i32)
              }
              frame 5 {
                w938 = FALSE  # no PTO
                w939 = FALSE  # not climbing
                w946 = FALSE  # pins in
                # "wait for the driver to start climbing"
                n316 = global read "Inputs_DriverStation.vi" "J1-RightTrigger"() -> (w935:dbl)
                n317 = Greater?(x=w935, y=0.2) -> (0:w933:bool)
                n318 = feedback #16(FALSE) -> (w940:bool)
                n319 = Select(t=TRUE, s=w933, f=w940) -> (s? t:f=w932:bool)
                n320 = feedback-in #16(w932) -> ()
                n321 = Increment(x=w944) -> (x+1=w945:i32)
                n322 = Select(t=w945, s=w932, f=w944) -> (s? t:f=w943:i32)
              }
              frame 6 {
                w954 = FALSE  # no PTO
                w955 = TRUE  # climbing
                w959 = FALSE  # pins in
                # "wait for elevator to pass PTO height"
                n323 = global read "SensorReadings.vi" "EncoderPos_Elevator"() -> (w947:dbl)
                n324 = Less Or Equal?(x=w947, y=w949) -> (x <= y?=w948:bool)
                n325 = Increment(x=w957) -> (x+1=w958:i32)
                n326 = Select(t=w958, s=w948, f=w957) -> (s? t:f=w956:i32)
              }
              frame 7 {
                w966 = TRUE  # PTO
                w967 = TRUE  # climbing
                w971 = FALSE  # pins in
                # "engage the PTO"
                n327 = Increment(x=w969) -> (x+1=w970:i32)
                n328 = Tick Count (ms)() -> (millisecond timer value=w960:u32)
                n329 = Select(t=w970, s=TRUE, f=w969) -> (s? t:f=w968:i32)
              }
              frame 8 {
                w985 = TRUE  # PTO
                w986 = TRUE  # climbing
                w990 = FALSE  # pins in
                # "timeout"
                # "ensure PTO is engaged"
                n330 = global read "SensorReadings.vi" "EncoderPos_Elevator"() -> (w980:dbl)
                n331 = Tick Count (ms)() -> (millisecond timer value=w976:u32)
                n332 = Less Or Equal?(x=w980, y=w979) -> (x <= y?=w978:bool)
                n333 = Subtract(x=w976, y=w973) -> (x-y=w975:u32)
                n334 = Greater?(x=w975, y=u32 1000) -> (0:w972:bool)
                n335 = Or(x=w972, y=w978) -> (x .or. y?=w977:bool)
                n336 = Increment(x=w988) -> (x+1=w989:i32)
                n337 = Select(t=w989, s=w977, f=w988) -> (s? t:f=w987:i32)
              }
              frame 9 {
                w995 = TRUE  # PTO
                w1002 = TRUE  # climbing
                w1001 = FALSE  # pins in
                # "wait for robot to be secure on HAB"
                n338 = global read "Inputs_DriverStation.vi" "Master_Safety_Override"() -> (w1003:bool)
                n339 = global read "SensorReadings.vi" "Robot On Ground"() -> (w991:bool)
                n340 = global read "Inputs_DriverStation.vi" "J1-Menu"() -> (w1004:bool)
                n341 = Or(x=w991, y=w1003) -> (x .or. y?=w999:bool)
                n342 = And(x=w1004, y=w999) -> (x .and. y?=w994:bool)
                n343 = Increment(x=w997) -> (x+1=w998:i32)
                n344 = Select(t=w998, s=w994, f=w997) -> (s? t:f=w996:i32)
              }
              frame 10 {
                w1010 = TRUE  # PTO
                w1016 = FALSE  # not climbing
                w1015 = FALSE  # pins in
                # "stop \"climbing\""
                n345 = Increment(x=w1012) -> (x+1=w1013:i32)
                n346 = Select(t=w1013, s=TRUE, f=w1012) -> (s? t:f=w1011:i32)
              }
              frame 11 {
                w1020 = TRUE  # PTO
                w1028 = FALSE  # not climbing
                w1027 = FALSE  # pins in
                # "wait to disengage PTO"
                n347 = Increment(x=w1024) -> (x+1=w1025:i32)
                n348 = Select(t=w1025, s=TRUE, f=w1024) -> (s? t:f=w1023:i32)
              }
              frame 12 {
                w1046 = FALSE  # no PTO
                w1050 = FALSE  # not climbing
                w1049 = FALSE  # pins in
                # "retract legs"
                n349 = global read "Inputs_DriverStation.vi" "J1-Menu"() -> (w1030:bool)
                n350 = Not(x=w1030) -> (.not. x?=w1031:bool)
                n351 = feedback #17(FALSE ("PTO")) -> (w1034:bool)
                n352 = Select(t=TRUE ("no PTO"), s=w1031, f=w1034) -> (s? t:f=w1029:bool)
                n353 = feedback-in #17(w1029) -> ()
                n354 = And(x=w1029, y=w1030) -> (x .and. y?=w1032:bool)
                n355 = feedback #18(FALSE ("PTO")) -> (w1038:bool)
                n356 = Select(t=TRUE ("no PTO"), s=w1032, f=w1038) -> (s? t:f=w1036:bool)
                n357 = feedback-in #18(w1036) -> ()
                n358 = Increment(x=w1041) -> (x+1=w1042:i32)
                n359 = Select(t=w1042, s=w1036, f=w1041) -> (s? t:f=w1040:i32)
              }
              frame 13 {
                w1051 = TRUE  # end of match
                w1056 = FALSE  # no PTO
                w1060 = FALSE  # not climbing
                w1059 = FALSE  # pins in
                # "turn off the elevator"
              }
            }
          }
          frame 2 {
            w1064 = 57.0  # Level 3 PTO Okay
            w1066 = 62.0  # Level 3 Start
            w1078 = 60.0  # Level 3 PTO
            # "Level 3 buddy climb sequence"
            n360 = case shown="1" w1075 {
              selector: w1075 -> [w1089 w1105 w1121 w1139 w1151 w1173 w1187 w1200 w1220 w1229 w1242 w1254 w1272 w1285]
              tunnel: [w1091 w1107 w1116 w1138 w1150 w1172 w1186 w1199 w1219 w1228 w1241 w1253 w1271 w1285] -> w1069
              tunnel: [w1088 w1095 w1114 w1136 w1153 w1165 w1182 w1191 w1205 w1231 w1244 w1256 w1278 w1288] -> w1076
              tunnel: w1077 -> [_ w1095 w1114 _ w1153 w1165 w1182 _ w1205 w1231 w1244 w1256 w1278 w1288]
              tunnel: [w1087 w1104 w1127 w1137 w1149 w1175 w1189 w1202 w1222 w1232 w1245 w1257 w1279 w1289] -> w1070
              tunnel: [w1080 w1094 w1110 w1130 w1143 w1159 _ w1194 w1215 _ _ _ _ _] -> w1068
              tunnel: w1078 -> [_ _ _ _ _ _ w1179 w1194 w1215 _ _ _ _ _]
              tunnel: [w1085 w1103 w1115 w1134 w1148 w1168 w1185 w1198 w1218 w1233 w1246 w1258 w1280 w1290] -> w1071
              tunnel: [w1084 w1102 w1113 w1133 w1147 w1167 w1184 w1197 w1217 w1227 w1240 w1251 w1276 w1286] -> w1072
              tunnel: [FALSE FALSE FALSE FALSE FALSE FALSE FALSE FALSE FALSE FALSE TRUE TRUE TRUE FALSE] -> w1073
              tunnel: w1074 -> [_ _ _ _ _ _ _ _ _ _ _ _ _ _]
              tunnel: ["release mantis" "wait for mantis to deploy" "wait for elevator to reach climb height" "lock mantis" "confirm mantis lock" "wait for the driver to start climbing" "wait for elevator to pass PTO height" "engage the PTO" "ensure PTO is engaged" "wait for the robot to be on HAB" "stop climbing" "wait to disengage PTO" "retract the legs after confirm " "elevator powered down"] -> w1067
              tunnel: w1066 -> [_ _ w1110 w1130 w1143 w1159 _ _ _ _ _ _ _ _]
              tunnel: [-1.0 ("y") -1.0 ("y") -1.0 ("y") -1.0 ("y") -1.0 ("y") -1.0 ("y") -0.05 ("y") -0.05 ("y") -0.05 ("y") -1.0 ("y") -1.0 ("y") -1.0 ("y") -1.0 ("y") -1.0 ("y")] -> w1065
              tunnel: w1064 -> [_ _ _ _ _ _ _ _ w1211 _ _ _ _ _]
              tunnel: [_ _ _ _ _ _ _ _ _ _ _ _ _ w1282] -> w1063
              tunnel: w1062 -> [w1080 w1094 _ _ _ _ _ _ _ _ _ _ _ _]
              tunnel: [w1079 w1092 w1108 w1128 w1141 w1157 w1176 w1190 w1203 w1223 w1235 w1247 w1259 w1281] -> w1061
              frame 0, Default {
                w1079 = FALSE  # foot retracted
                w1084 = FALSE  # no PTO
                w1085 = FALSE  # not climbing
                w1087 = TRUE  # pins out
                # "release mantis pins and command to climb height"
                n361 = Increment(x=w1089) -> (x+1=w1090:i32)
                n362 = Select(t=w1090, s=TRUE, f=w1089) -> (s? t:f=w1091:i32)
                n363 = Tick Count (ms)() -> (millisecond timer value=w1088:u32)
              }
              frame 1 {
                w1092 = FALSE  # foot retracted
                w1102 = FALSE  # no PTO
                w1103 = FALSE  # not climbing
                w1104 = TRUE  # pins out
                # "wait for mantis to deploy"
                n364 = Tick Count (ms)() -> (millisecond timer value=w1098:u32)
                n365 = Subtract(x=w1098, y=w1095) -> (x-y=w1097:u32)
                n366 = Greater?(x=w1097, y=u32 250) -> (0:w1093:bool)
                n367 = Increment(x=w1105) -> (x+1=w1106:i32)
                n368 = Select(t=w1106, s=w1093, f=w1105) -> (s? t:f=w1107:i32)
              }
              frame 2 {
                w1108 = FALSE  # foot retracted
                w1113 = FALSE  # no PTO
                w1115 = FALSE  # not climbing
                w1127 = TRUE  # pins out
                # "wait for elevator to start moving\nand then stop moving"
                # "wait for elevator to reach climb position"
                n369 = global read "RobotStates.vi" "Elevator Moving"() -> (w1119:bool)
                n370 = call "RisingEdgeTrigger.vi"("Raw Signal"=w1119) -> ("Trigger"=w1126:bool)
                n371 = Not(x=w1119) -> (.not. x?=w1118:bool)
                n372 = feedback #19(FALSE) -> (w1124:bool)
                n373 = Select(t=TRUE, s=w1126, f=w1124) -> (s? t:f=w1120:bool)
                n374 = feedback-in #19(w1120) -> ()
                n375 = And(x=w1120, y=w1118) -> (x .and. y?=w1117:bool)
                n376 = Increment(x=w1121) -> (x+1=w1122:i32)
                n377 = Select(t=w1122, s=w1117, f=w1121) -> (s? t:f=w1116:i32)
              }
              frame 3 {
                w1128 = FALSE  # foot retracted
                w1133 = FALSE  # no PTO
                w1134 = FALSE  # not climbing
                w1137 = FALSE  # pins in
                # "lock mantis pins"
                n378 = Increment(x=w1139) -> (x+1=w1140:i32)
                n379 = Tick Count (ms)() -> (millisecond timer value=w1136:u32)
                n380 = Select(t=w1140, s=TRUE, f=w1139) -> (s? t:f=w1138:i32)
              }
              frame 4 {
                w1141 = FALSE  # foot retracted
                w1147 = FALSE  # no PTO
                w1148 = FALSE  # not climbing
                w1149 = FALSE  # pins in
                # "wait for mantis legs to lock"
                n381 = Tick Count (ms)() -> (millisecond timer value=w1156:u32)
                n382 = Subtract(x=w1156, y=w1153) -> (x-y=w1155:u32)
                n383 = Greater?(x=w1155, y=u32 500) -> (0:w1145:bool)
                n384 = Increment(x=w1151) -> (x+1=w1152:i32)
                n385 = Select(t=w1152, s=w1145, f=w1151) -> (s? t:f=w1150:i32)
              }
              frame 5 {
                w1157 = FALSE  # foot retracted
                w1167 = FALSE  # no PTO
                w1168 = FALSE  # not climbing
                w1175 = FALSE  # pins in
                # "wait for the driver to start climbing"
                n386 = global read "Inputs_DriverStation.vi" "J1-RightTrigger"() -> (w1164:dbl)
                n387 = Greater?(x=w1164, y=0.2) -> (0:w1162:bool)
                n388 = feedback #20(FALSE) -> (w1169:bool)
                n389 = Select(t=TRUE, s=w1162, f=w1169) -> (s? t:f=w1161:bool)
                n390 = feedback-in #20(w1161) -> ()
                n391 = Increment(x=w1173) -> (x+1=w1174:i32)
                n392 = Select(t=w1174, s=w1161, f=w1173) -> (s? t:f=w1172:i32)
              }
              frame 6 {
                w1176 = FALSE  # foot retracted
                w1184 = FALSE  # no PTO
                w1185 = TRUE  # climbing
                w1189 = FALSE  # pins in
                # "wait for elevator to pass PTO height"
                n393 = global read "SensorReadings.vi" "EncoderPos_Elevator"() -> (w1177:dbl)
                n394 = Less Or Equal?(x=w1177, y=w1179) -> (x <= y?=w1178:bool)
                n395 = Increment(x=w1187) -> (x+1=w1188:i32)
                n396 = Select(t=w1188, s=w1178, f=w1187) -> (s? t:f=w1186:i32)
              }
              frame 7 {
                w1190 = FALSE  # foot retracted
                w1197 = TRUE  # PTO
                w1198 = TRUE  # climbing
                w1202 = FALSE  # pins in
                # "engage the PTO"
                n397 = Increment(x=w1200) -> (x+1=w1201:i32)
                n398 = Tick Count (ms)() -> (millisecond timer value=w1191:u32)
                n399 = Select(t=w1201, s=TRUE, f=w1200) -> (s? t:f=w1199:i32)
              }
              frame 8 {
                w1203 = FALSE  # foot retracted
                w1217 = TRUE  # PTO
                w1218 = TRUE  # climbing
                w1222 = FALSE  # pins in
                # "timeout"
                # "ensure PTO is engaged"
                n400 = global read "SensorReadings.vi" "EncoderPos_Elevator"() -> (w1212:dbl)
                n401 = Tick Count (ms)() -> (millisecond timer value=w1208:u32)
                n402 = Less Or Equal?(x=w1212, y=w1211) -> (x <= y?=w1210:bool)
                n403 = Subtract(x=w1208, y=w1205) -> (x-y=w1207:u32)
                n404 = Greater?(x=w1207, y=u32 1000) -> (0:w1204:bool)
                n405 = Or(x=w1204, y=w1210) -> (x .or. y?=w1209:bool)
                n406 = Increment(x=w1220) -> (x+1=w1221:i32)
                n407 = Select(t=w1221, s=w1209, f=w1220) -> (s? t:f=w1219:i32)
              }
              frame 9 {
                w1223 = TRUE  # foot deployed
                w1227 = TRUE  # PTO
                w1233 = TRUE  # climbing
                w1232 = FALSE  # pins in
                # "wait for robot to be secure on HAB"
                n408 = global read "Inputs_DriverStation.vi" "J1-Menu"() -> (w1234:bool)
                n409 = Increment(x=w1229) -> (x+1=w1230:i32)
                n410 = Select(t=w1230, s=w1234, f=w1229) -> (s? t:f=w1228:i32)
              }
              frame 10 {
                w1235 = TRUE  # foot deployed
                w1240 = TRUE  # PTO
                w1246 = TRUE  # climbing
                w1245 = FALSE  # pins in
                # "******"
                # "stop \"climbing\""
                n411 = Increment(x=w1242) -> (x+1=w1243:i32)
                n412 = Select(t=w1243, s=TRUE, f=w1242) -> (s? t:f=w1241:i32)
              }
              frame 11 {
                w1247 = TRUE  # foot deployed
                w1251 = TRUE  # PTO
                w1258 = TRUE  # climbing
                w1257 = FALSE  # pins in
                # "******"
                # "wait to disengage PTO"
                n413 = Increment(x=w1254) -> (x+1=w1255:i32)
                n414 = Select(t=w1255, s=TRUE, f=w1254) -> (s? t:f=w1253:i32)
              }
              frame 12 {
                w1259 = TRUE  # foot deployed
                w1276 = FALSE  # no PTO
                w1280 = TRUE  # climbing
                w1279 = FALSE  # pins in
                # "*******"
                # "retract legs"
                n415 = global read "Inputs_DriverStation.vi" "J1-Menu"() -> (w1261:bool)
                n416 = Not(x=w1261) -> (.not. x?=w1262:bool)
                n417 = feedback #21(FALSE ("PTO")) -> (w1265:bool)
                n418 = Select(t=TRUE ("no PTO"), s=w1262, f=w1265) -> (s? t:f=w1260:bool)
                n419 = feedback-in #21(w1260) -> ()
                n420 = And(x=w1260, y=w1261) -> (x .and. y?=w1263:bool)
                n421 = feedback #22(FALSE ("PTO")) -> (w1269:bool)
                n422 = Select(t=TRUE ("no PTO"), s=w1263, f=w1269) -> (s? t:f=w1267:bool)
                n423 = feedback-in #22(w1267) -> ()
                n424 = Increment(x=w1272) -> (x+1=w1273:i32)
                n425 = Select(t=w1273, s=w1267, f=w1272) -> (s? t:f=w1271:i32)
              }
              frame 13 {
                w1281 = TRUE  # foot deployed
                w1282 = TRUE  # end of match
                w1286 = FALSE  # no PTO
                w1290 = TRUE  # climbing
                w1289 = FALSE  # pins in
                # "turn off the elevator"
              }
            }
          }
        }
      }
      n426 = feedback-in #8(w537) -> ()
      n427 = global write "RobotStates.vi" "Climb Sequence"(w532) -> ()
    }
  }
  "Target Elevator Position" <- w58
  "Target Vacuum Pump Power" <- w55
  n428 = feedback-in #5(w20) -> ()
  n429 = global write "RobotStates.vi" "Climb Sequence String"(w8) -> ()
  n430 = global write "SensorReadings.vi" "LimeLight In Range"(w5) -> ()
  n431 = global write "RobotStates.vi" "Climber Foot State"(w2) -> ()
  n432 = global write "SensorReadings.vi" "At HAB Height"(w9) -> ()
  n433 = global write "RobotStates.vi" "Max Climb Power"(w7) -> ()
  n434 = global write "RobotStates.vi" "End of Match"(w6) -> ()
  n435 = global write "RobotStates.vi" "PTO State"(w13) -> ()
  n436 = global write "RobotStates.vi" "Climb Started"(w14) -> ()
  n437 = global write "RobotStates.vi" "Climber Mantis State"(w1) -> ()
  n438 = global write "RobotStates.vi" "Upper Valve State"(w52) -> ()
  n439 = global write "RobotStates.vi" "Lower Valve State"(w51) -> ()
  n440 = global write "RobotStates.vi" "CARGO Intake Allowed"(w60) -> ()
  n441 = global write "RobotStates.vi" "CARGO Arm"(w59) -> ()
  n442 = global write "RobotStates.vi" "HATCH Arm"(w57) -> ()
  n443 = global write "RobotStates.vi" "HATCH Ejection Allowed"(w56) -> ()
  n444 = global read "Inputs_DriverStation.vi" "J1-View"() -> (w31:bool)
  n445 = Equal?(x=w29, y="Elevator_Stow") -> (x = y?=w45:bool)
  n446 = Equal?(x=w29, y="Cargo_Ground") -> (x = y?=w44:bool)
  n447 = Equal?(x=w29, y="Cargo_Feeder") -> (x = y?=w43:bool)
  n448 = Equal?(x=w29, y="Hatch_Ground") -> (x = y?=w42:bool)
  n449 = Equal?(x=w29, y="Hatch_Feeder") -> (x = y?=w41:bool)
  n450 = Equal?(x=w29, y="Climb") -> (x = y?=w40:bool)
  n451 = Compound Arithmetic op=OR(w45, w44, w43, w42, w41, w40, w31) -> (w37:bool)
  n452 = Not(x=w37) -> (.not. x?=w36:bool)
  n453 = while {
    shift-right: [w1295] -> w30
    shift-left: _ -> [w1296]
    tunnel: w36 -> [w1294]
    shift-right: [w1293] -> _
    shift-left: _ -> [w1292]
    tunnel: w29 -> [w1291]
    tunnel: [w1291] -> w28
    stop <- TRUE stop-if-true
    n454 = case shown="True" w1294 {
      tunnel: w1296 -> [_ w1303]
      tunnel: [0 w1302] -> w1295
      tunnel: [w1298 w1301] -> w1293
      tunnel: w1292 -> [w1298 w1300]
      frame False {
        # "stow, ground pickup, or feeder station"
      }
      frame True {
        # "rocket are cargo ship"
        n455 = case shown="1" w1303 {
          selector: w1303 -> [w1306 w1314 w1328 w1339 w1343 _]
          tunnel: [w1305 w1316 w1323 w1340 w1342 0 ("t")] -> w1302
          tunnel: [w1304 w1313 w1321 w1333 w1341 w1349] -> w1301
          tunnel: w1300 -> [w1304 _ w1321 _ w1341 w1349]
          frame 0, Default {
            # "wait for driver to start release"
            n456 = global read "Inputs_DriverStation.vi" "J1-LeftTrigger"() -> (w1309:dbl)
            n457 = Greater?(x=w1309, y=0.75) -> (0:w1307:bool)
            n458 = Increment(x=w1306) -> (x+1=w1310:i32)
            n459 = Select(t=w1310, s=w1307, f=w1306) -> (s? t:f=w1305:i32)
          }
          frame 1 {
            # "check for game piece release"
            n460 = global read "SensorReadings.vi" "Hatch Captured"() -> (w1319:bool)
            n461 = global read "SensorReadings.vi" "Cargo Captured"() -> (w1318:bool)
            n462 = Not(x=w1318) -> (.not. x?=w1312:bool)
            n463 = Not(x=w1319) -> (.not. x?=w1311:bool)
            n464 = Or(x=w1311, y=w1312) -> (x .or. y?=w1317:bool)
            n465 = Increment(x=w1314) -> (x+1=w1315:i32)
            n466 = Tick Count (ms)() -> (millisecond timer value=w1313:u32)
            n467 = Select(t=w1315, s=w1317, f=w1314) -> (s? t:f=w1316:i32)
          }
          frame 2 {
            # "***200"
            # "check to see if game piece actually gone"
            n468 = global read "SensorReadings.vi" "Hatch Captured"() -> (w1325:bool)
            n469 = global read "SensorReadings.vi" "Cargo Captured"() -> (w1326:bool)
            n470 = Tick Count (ms)() -> (millisecond timer value=w1332:u32)
            n471 = Subtract(x=w1332, y=w1321) -> (x-y=w1331:u32)
            n472 = Greater?(x=w1331, y=u32 0) -> (0:w1329:bool)
            n473 = Or(x=w1325, y=w1326) -> ()  [unwired: 1 out]
            n474 = Increment(x=w1328) -> (x+1=w1327:i32)
            n475 = Select(t=w1327, s=w1329, f=w1328) -> (s? t:f=w1324:i32)
            n476 = Select(t=0, s=FALSE, f=w1324) -> (s? t:f=w1323:i32)
          }
          frame 3 {
            # "wait for driver to release trigger"
            n477 = global read "Inputs_DriverStation.vi" "J1-LeftTrigger"() -> (w1337:dbl)
            n478 = Greater?(x=w1337, y=0.1) -> (0:w1335:bool)
            n479 = Not(x=w1335) -> (.not. x?=w1334:bool)
            n480 = Increment(x=w1339) -> (x+1=w1338:i32)
            n481 = Select(t=w1338, s=w1334, f=w1339) -> (s? t:f=w1340:i32)
            n482 = Tick Count (ms)() -> (millisecond timer value=w1333:u32)
          }
          frame 4 {
            # "safety wait"
            n483 = Tick Count (ms)() -> (millisecond timer value=w1348:u32)
            n484 = Subtract(x=w1348, y=w1341) -> (x-y=w1347:u32)
            n485 = Greater?(x=w1347, y=u32 50) -> (0:w1345:bool)
            n486 = Increment(x=w1343) -> (x+1=w1344:i32)
            n487 = Select(t=w1344, s=w1345, f=w1343) -> (s? t:f=w1342:i32)
          }
          frame 5 {
            # "trigger auto stow"
            n488 = global write "RobotStates.vi" "Auto Stow"(TRUE) -> ()
          }
        }
      }
    }
  }
  "Elevator State Out" <- w28
  n489 = global write "RobotStates.vi" "Auto Stow Sequence"(w30) -> ()
